vi "FTW-Endpoint-Receive-Worker.vi"(0 "FTW Endpoint":refnum<class "FTW-Endpoint.lvclass">, 5 "Address":string) -> ()   [LabVIEW 2013, in "FTW-Endpoint.lvclass"]
uses:
  FTW-Endpoint.lvclass
  FTW-Endpoint.lvclass/FTW-Endpoint.ctl
panel:
  out "connected":bool
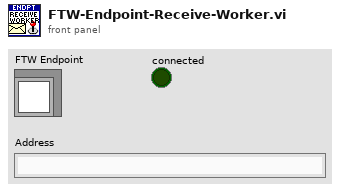
[diagram p1: front panel]
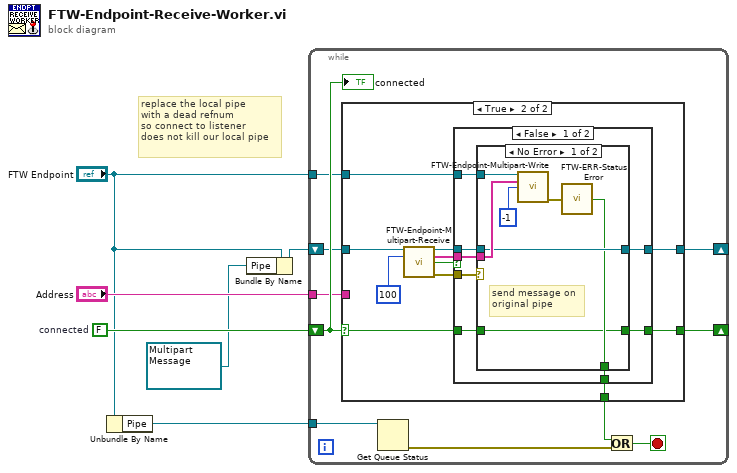
[diagram p0: block diagram]
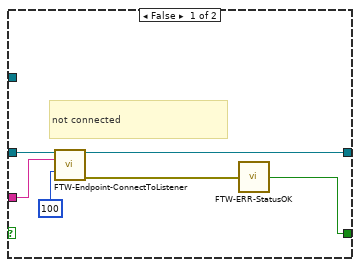
[diagram p2: hidden frame]
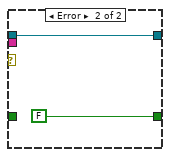
[diagram p3: hidden frame]
diagram:
  w6 = FALSE  # connected
  # "replace the local pipe\nwith a dead refnum\nso connect to listener\ndoes not kill our local pipe"
  n1 = Unbundle By Name("FTW Endpoint") -> ("Pipe"=w4:refnum<queue>)
  n2 = Bundle By Name(cluster="FTW Endpoint", "Pipe"=refnum<queue> refnum) -> (w2:refnum<class "FTW-Endpoint.lvclass">)
  n3 = while {
    shift-right: [w13] -> _
    shift-left: w6 -> [w16]
    shift-right: [w14] -> _
    shift-left: w2 -> [w10]
    tunnel: "Address" -> [w15]
    tunnel: w4 -> [w12]
    tunnel: "FTW Endpoint" -> [w7]
    stop <- w9 stop-if-true
    n4 = case shown="True" w16 {
      selector: w16 -> [_ w30]
      tunnel: w15 -> [w22 _]
      tunnel: [w17 w32] -> w14
      tunnel: [w21 w31] -> w13
      tunnel: w10 -> [w18 w33]
      tunnel: [_ w24] -> w8
      tunnel: w7 -> [_ w25]
      frame False {
        # "not connected"
        n5 = call-dynamic "FTW-Endpoint-ConnectToListener.vi"("FTW-Endpoint In"=w18, "Address"=w22, "Timeout"=100) -> ("FTW-Endpoint Out"=w17:refnum<class "FTW-Endpoint.lvclass">, "error out"=w20:errorcluster)  [unwired: 10 in, 1 out]
        n6 = call "FTW-ERR-StatusOK.vi"("error to check"=w20) -> ("Status OK?"=w21:bool)
      }
      frame True {
        n7 = call-dynamic "FTW-Endpoint-Multipart-Receive.vi"("FTW Endpoint"=w33, "Timeout"=100) -> ("FTW Endpoint out"=w29:refnum<class "FTW-Endpoint.lvclass">, "Message Received"=w26:string[], "Timed out?"=w23:bool, "error out"=w28:errorcluster)  [unwired: 10 in]
        n8 = case shown="False" w23 {
          tunnel: [w41 w52] -> w32
          tunnel: [w40 w51] -> w31
          tunnel: w30 -> [w39 w51]
          tunnel: w29 -> [w38 w52]
          tunnel: w28 -> [w37 _]
          tunnel: w26 -> [w36 _]
          tunnel: w25 -> [w35 _]
          tunnel: [w34 _] -> w24
          frame False {
            n9 = case shown="No Error" w37 {
              tunnel: [w45 w50] -> w41
              tunnel: [w42 FALSE ("Status OK?")] -> w40
              tunnel: w39 -> [w42 _]
              tunnel: w38 -> [w45 w50]
              tunnel: w36 -> [w48 _]
              tunnel: w35 -> [w46 _]
              tunnel: [w43 _] -> w34
              frame No Error {
                # "send message on\noriginal pipe"
                n10 = call-dynamic "FTW-Endpoint-Multipart-Write.vi"("FTW Endpoint"=w46, "Multipart Message"=w48, "Timeout"=-1) -> ("error out"=w44:errorcluster)  [unwired: 10 in, 2 out]
                n11 = call "FTW-ERR-StatusError.vi"("error to check"=w44) -> ("Error?"=w43:bool)
              }
              frame Error {
              }
            }
          }
          frame True {
          }
        }
      }
    }
    n12 = Get Queue Status(queue=w12) -> (error out=w11:errorcluster)  [unwired: 2 in, 7 out]
    n13 = Or(x=w8, y=w11) -> (x .or. y?=w9:bool)
    "connected" <- w16
  }
